vi "Test_CommonTypes_ValuesOK.vi"(8 "error in (no error)":errorcluster, 11 "TestCase in":refnum<class "TestVariantExtensions.lvclass">) -> (0 "error out":errorcluster, 3 "TestCase out":refnum<class "TestVariantExtensions.lvclass">)   [LabVIEW 2015, in "TestVariantExtensions.lvclass"]
uses:
  TestVariantExtensions.lvclass
  Scalar Data to String.vi
  <vilib>/Utility/Data Type/Get Type Information.vi
  <vilib>/addons/_JKI Toolkits/VI Tester/TestCase.llb/TestCase.lvclass
  VariantExtensions.lvlib
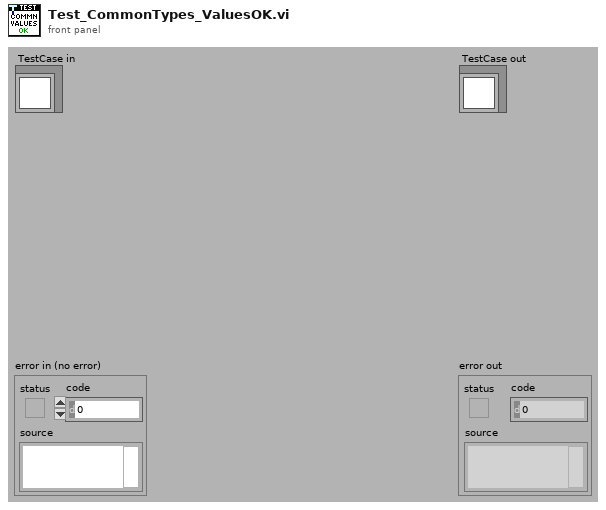
[diagram p1: front panel]
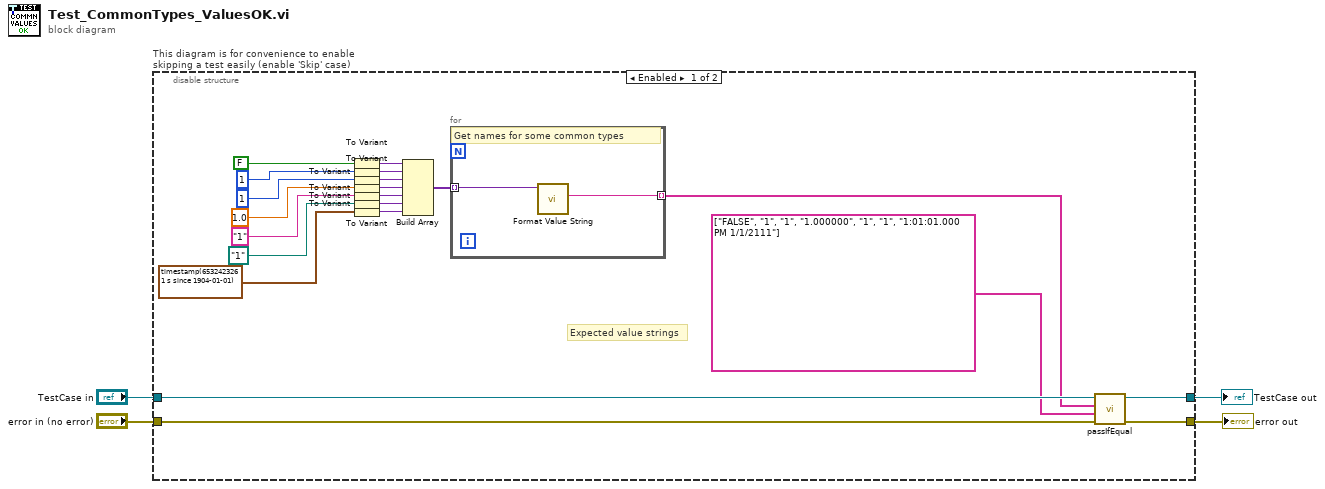
[diagram p0: block diagram]
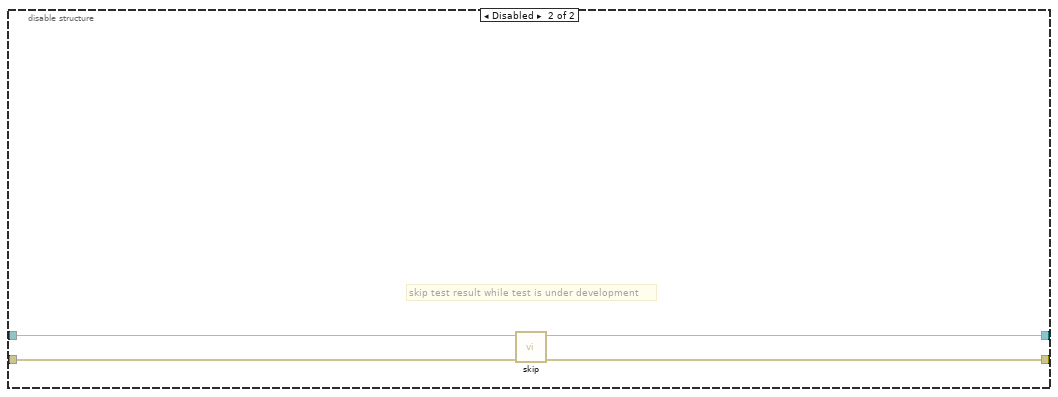
[diagram p2: hidden frame]
diagram:
  n1 = disable-structure "This diagram is for convenience to enable skipping a test easily (enable 'Skip' case)" shown="Enabled" {
    disable-tunnel: "TestCase in" -> [w25 w31]
    disable-tunnel: [w24 w29] -> w1
    disable-tunnel: [w23 w30] -> w3
    disable-tunnel: "error in (no error)" -> [w22 w28]
    frame Enabled {
      # "Expected value strings"
      n2 = To Variant(anything=FALSE) -> (Variant=w6:variant)
      n3 = To Variant(anything=u32 1) -> (Variant=w21:variant)
      n4 = To Variant(anything=1) -> (Variant=w20:variant)
      n5 = To Variant(anything=1.0) -> (Variant=w19:variant)
      n6 = To Variant(anything="1") -> (Variant=w18:variant)
      n7 = To Variant(anything=path "1") -> (Variant=w17:variant)
      n8 = To Variant(anything=timestamp(6532423261 s since 1904-01-01)) -> (Variant=w16:variant)
      n9 = Build Array(w6, w21, w20, w19, w18, w17, w16) -> (w9:variant[])
      n10 = for {
        tunnel: [w27] -> w8 mode=indexing
        tunnel: w9 -> [w26] mode=indexing
        # "Get names for some common types"
        n11 = call "Format Value String.vi"("Data"=w26) -> ("Value as String"=w27:string)  [unwired: 9 in, 1 out]
      }
      n12 = call-dynamic "passIfEqual.vi"("error in (no error)"=w22, "y"=string[] ["FALSE", "1", "1", "1.000000", "1", "1", "1:01:01.000 PM 1/1/2111"] ("Array"), "x"=w8, "TestCase in"=w25) -> ("error out"=w23:errorcluster, "TestCase out"=w24:refnum<class "TestVariantExtensions.lvclass">)  [unwired: 6 in]
    }
    frame Disabled {
      # "skip test result while test is under development"
      n13 = call <vilib>:"skip.vi"("error in (no error)"=w28, "TestCase in"=w31) -> ("error out"=w30:errorcluster, "TestCase out"=w29:refnum<class "TestVariantExtensions.lvclass">)  [unwired: 8 in]
    }
  }
  "error out" <- w3
  "TestCase out" <- w1
